vi "CLSUIP_GetContainingLVClass.vi"(8 "error in (no error)":errorcluster, 11 "Member VI":refnum<vi>) -> (0 "error out":errorcluster, 2 "Containing LVClass":refnum<vi>, 3 "Member VI out":refnum<vi>)   [LabVIEW 2021, in "MemberVICreation.lvlib" / "VIRetooler.lvclass"]
uses:
  <resource>/Framework/Providers/LVClassLibrary/NewAccessors/VIRetooler/VIRetooler.lvclass
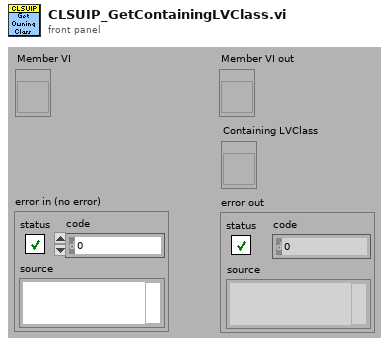
[diagram p1: front panel]
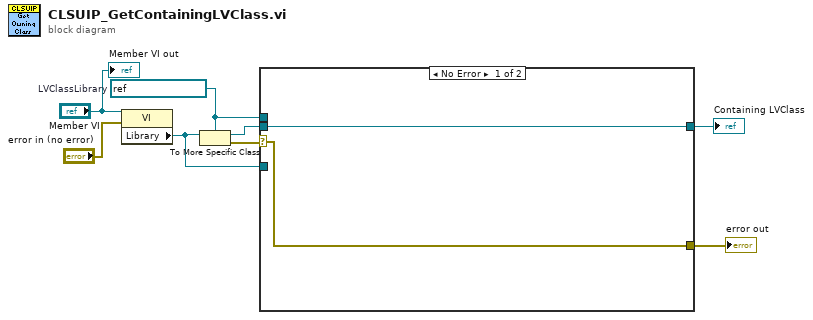
[diagram p0: block diagram]
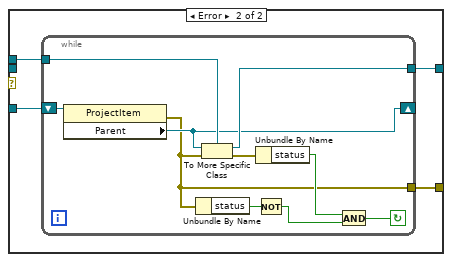
[diagram p2: hidden frame]
diagram:
  w4 = refnum<vi> refnum  # LVClassLibrary
  n1 = property class="VI"(reference="Member VI", error in="error in (no error)") -> ("Library"=w5:refnum<vi>)  [unwired: 2 out]
  n2 = To More Specific Class(target class=w4, reference=w5) -> (specific class reference=w6:refnum<vi>, error out=w8:errorcluster)  [unwired: 1 in]
  n3 = case shown="No Error" w8 {
    selector: w8 -> [w9 _]
    tunnel: [w10 w12] -> w7
    tunnel: w6 -> [w10 _]
    tunnel: w5 -> [_ w14]
    tunnel: w4 -> [_ w13]
    tunnel: [w9 w11] -> w2
    frame No Error {
    }
    frame Error {
      n4 = while {
        shift-right: [w16] -> _
        shift-left: w14 -> [w24]
        tunnel: w13 -> [w23]
        tunnel: [w17] -> w12
        tunnel: [w15] -> w11
        stop <- w18 continue-if-true
        n5 = property class="ProjectItem"(reference=w24) -> (error out=w15:errorcluster, "Parent"=w16:refnum<vi>)  [unwired: 1 in, 1 out]
        n6 = Unbundle By Name(w15) -> ("status"=w21:bool)
        n7 = To More Specific Class(target class=w23, reference=w16, error in=w15) -> (specific class reference=w17:refnum<vi>, error out=w22:errorcluster)
        n8 = Unbundle By Name(w22) -> ("status"=w19:bool)
        n9 = Not(x=w21) -> (.not. x?=w20:bool)
        n10 = And(x=w19, y=w20) -> (x .and. y?=w18:bool)
      }
    }
  }
  "Containing LVClass" <- w7
  "error out" <- w2
  "Member VI out" <- "Member VI"
